vi "CRYCal Correction.vi"(4 "Calibration Response Cluster":T1={"Calibration"={"Calibration Step Name"="", "Device"="", "Correction Curve Name"="", "Equalization Curve Name"="", "Sensitivity Curve Name"="", "Corr Folder and File"="", "EQ Folder and File"="", "Sens Folder and File"="", "Corr Step size"=0, "EQ Step size"=0, "Input"=FALSE, "Last Cal Date (sec)"=timestamp(0 s since 1904-01-01), "Cha Name"="", "Corr Curve Found"=FALSE, "EQ Curve Found"=FALSE, "Sens Curve Found"=FALSE, "Signal Type"="", "Calibrated Device"="", "Hz"=0}, "Corr Curve"={"Name"="", "Curve"=[], "X data"=1, "Y data"=1, "Z data"=1, "X axis"=0, "Y axis"=1, "Z axis"=1, "X unit"="Hz", "Y unit"="", "Z unit"="deg.", "X dB ref"=1.0, "Y dB ref"=1.0, "Z dB ref"=1.0, "single val"=FALSE, "protected"=FALSE, "display X"=TRUE, "display Y"=TRUE, "display Z"=TRUE, "Test Info"="", "Step No."=0, "Plot Settings"={"Color"=0, "Interpolation"=0, "Point Style"=0, "Line Style"=0, "Point Color"=0, "Line Width"=0, "Bar Plot Style"=0, "Fill To"=0}, "AutoProtect"=FALSE}, "EQ Curve"={"Name"="", "Curve"=[], "X data"=1, "Y data"=1, "Z data"=1, "X axis"=0, "Y axis"=1, "Z axis"=1, "X unit"="Hz", "Y unit"="", "Z unit"="deg.", "X dB ref"=1.0, "Y dB ref"=1.0, "Z dB ref"=1.0, "single val"=FALSE, "protected"=FALSE, "display X"=TRUE, "display Y"=TRUE, "display Z"=TRUE, "Test Info"="", "Step No."=0, "Plot Settings"={"Color"=0, "Interpolation"=0, "Point Style"=0, "Line Style"=0, "Point Color"=0, "Line Width"=0, "Bar Plot Style"=0, "Fill To"=0}, "AutoProtect"=FALSE}, "Sens Curve"={"Name"="", "Curve"=[], "X data"=1, "Y data"=1, "Z data"=1, "X axis"=0, "Y axis"=1, "Z axis"=1, "X unit"="Hz", "Y unit"="", "Z unit"="deg.", "X dB ref"=1.0, "Y dB ref"=1.0, "Z dB ref"=1.0, "single val"=FALSE, "protected"=FALSE, "display X"=TRUE, "display Y"=TRUE, "display Z"=TRUE, "Test Info"="", "Step No."=0, "Plot Settings"={"Color"=0, "Interpolation"=0, "Point Style"=0, "Line Style"=0, "Point Color"=0, "Line Width"=0, "Bar Plot Style"=0, "Fill To"=0}, "AutoProtect"=FALSE}} {"Sens Curve"."Z data" items=["dB", "Lin"]; "Sens Curve"."X data" items=["dB", "Lin"]; "Sens Curve"."Y data" items=["dB", "Lin"]; "Sens Curve"."Z dB ref" format="%.1f"; "Sens Curve"."Z axis" items=["Log", "Lin"]; "Sens Curve"."X dB ref" format="%.1f"; "Sens Curve"."X axis" items=["Log", "Lin"]; "Sens Curve"."Y axis" items=["Log", "Lin"]; "Sens Curve"."Y dB ref" format="%.1f"; "Sens Curve"."Curve"."z" format="%.2f"; "Sens Curve"."Curve"."y" format="%.2f"; "Sens Curve"."Curve"."x" format="%.2f"; "EQ Curve"."Z data" items=["dB", "Lin"]; "EQ Curve"."X data" items=["dB", "Lin"]; "EQ Curve"."Y data" items=["dB", "Lin"]; "EQ Curve"."Z dB ref" format="%.1f"; "EQ Curve"."Z axis" items=["Log", "Lin"]; "EQ Curve"."X dB ref" format="%.1f"; "EQ Curve"."X axis" items=["Log", "Lin"]; "EQ Curve"."Y axis" items=["Log", "Lin"]; "EQ Curve"."Y dB ref" format="%.1f"; "EQ Curve"."Curve"."z" format="%.2f"; "EQ Curve"."Curve"."y" format="%.2f"; "EQ Curve"."Curve"."x" format="%.2f"; "Corr Curve"."Z data" items=["dB", "Lin"]; "Corr Curve"."X data" items=["dB", "Lin"]; "Corr Curve"."Y data" items=["dB", "Lin"]; "Corr Curve"."Z dB ref" format="%.1f"; "Corr Curve"."Z axis" items=["Log", "Lin"]; "Corr Curve"."X dB ref" format="%.1f"; "Corr Curve"."X axis" items=["Log", "Lin"]; "Corr Curve"."Y axis" items=["Log", "Lin"]; "Corr Curve"."Y dB ref" format="%.1f"; "Corr Curve"."Curve"."z" format="%.2f"; "Corr Curve"."Curve"."y" format="%.2f"; "Corr Curve"."Curve"."x" format="%.2f"; "Calibration"."EQ Step size" items=["R10", "R20", "R40", "R80", "User"]; "Calibration"."Corr Step size" items=["R10", "R20", "R40", "R80", "User"]}, 6 "Calibration Stimulus Cluster":T1={"Calibration"={"Calibration Step Name"="", "Device"="", "Correction Curve Name"="", "Equalization Curve Name"="", "Sensitivity Curve Name"="", "Corr Folder and File"="", "EQ Folder and File"="", "Sens Folder and File"="", "Corr Step size"=0, "EQ Step size"=0, "Input"=FALSE, "Last Cal Date (sec)"=timestamp(0 s since 1904-01-01), "Cha Name"="", "Corr Curve Found"=FALSE, "EQ Curve Found"=FALSE, "Sens Curve Found"=FALSE, "Signal Type"="", "Calibrated Device"="", "Hz"=0}, "Corr Curve"={"Name"="", "Curve"=[], "X data"=1, "Y data"=1, "Z data"=1, "X axis"=0, "Y axis"=1, "Z axis"=1, "X unit"="Hz", "Y unit"="", "Z unit"="deg.", "X dB ref"=1.0, "Y dB ref"=1.0, "Z dB ref"=1.0, "single val"=FALSE, "protected"=FALSE, "display X"=TRUE, "display Y"=TRUE, "display Z"=TRUE, "Test Info"="", "Step No."=0, "Plot Settings"={"Color"=0, "Interpolation"=0, "Point Style"=0, "Line Style"=0, "Point Color"=0, "Line Width"=0, "Bar Plot Style"=0, "Fill To"=0}, "AutoProtect"=FALSE}, "EQ Curve"={"Name"="", "Curve"=[], "X data"=1, "Y data"=1, "Z data"=1, "X axis"=0, "Y axis"=1, "Z axis"=1, "X unit"="Hz", "Y unit"="", "Z unit"="deg.", "X dB ref"=1.0, "Y dB ref"=1.0, "Z dB ref"=1.0, "single val"=FALSE, "protected"=FALSE, "display X"=TRUE, "display Y"=TRUE, "display Z"=TRUE, "Test Info"="", "Step No."=0, "Plot Settings"={"Color"=0, "Interpolation"=0, "Point Style"=0, "Line Style"=0, "Point Color"=0, "Line Width"=0, "Bar Plot Style"=0, "Fill To"=0}, "AutoProtect"=FALSE}, "Sens Curve"={"Name"="", "Curve"=[], "X data"=1, "Y data"=1, "Z data"=1, "X axis"=0, "Y axis"=1, "Z axis"=1, "X unit"="Hz", "Y unit"="", "Z unit"="deg.", "X dB ref"=1.0, "Y dB ref"=1.0, "Z dB ref"=1.0, "single val"=FALSE, "protected"=FALSE, "display X"=TRUE, "display Y"=TRUE, "display Z"=TRUE, "Test Info"="", "Step No."=0, "Plot Settings"={"Color"=0, "Interpolation"=0, "Point Style"=0, "Line Style"=0, "Point Color"=0, "Line Width"=0, "Bar Plot Style"=0, "Fill To"=0}, "AutoProtect"=FALSE}} {"Sens Curve"."Z data" items=["dB", "Lin"]; "Sens Curve"."X data" items=["dB", "Lin"]; "Sens Curve"."Y data" items=["dB", "Lin"]; "Sens Curve"."Z dB ref" format="%.1f"; "Sens Curve"."Z axis" items=["Log", "Lin"]; "Sens Curve"."X dB ref" format="%.1f"; "Sens Curve"."X axis" items=["Log", "Lin"]; "Sens Curve"."Y axis" items=["Log", "Lin"]; "Sens Curve"."Y dB ref" format="%.1f"; "Sens Curve"."Curve"."z" format="%.2f"; "Sens Curve"."Curve"."y" format="%.2f"; "Sens Curve"."Curve"."x" format="%.2f"; "EQ Curve"."Z data" items=["dB", "Lin"]; "EQ Curve"."X data" items=["dB", "Lin"]; "EQ Curve"."Y data" items=["dB", "Lin"]; "EQ Curve"."Z dB ref" format="%.1f"; "EQ Curve"."Z axis" items=["Log", "Lin"]; "EQ Curve"."X dB ref" format="%.1f"; "EQ Curve"."X axis" items=["Log", "Lin"]; "EQ Curve"."Y axis" items=["Log", "Lin"]; "EQ Curve"."Y dB ref" format="%.1f"; "EQ Curve"."Curve"."z" format="%.2f"; "EQ Curve"."Curve"."y" format="%.2f"; "EQ Curve"."Curve"."x" format="%.2f"; "Corr Curve"."Z data" items=["dB", "Lin"]; "Corr Curve"."X data" items=["dB", "Lin"]; "Corr Curve"."Y data" items=["dB", "Lin"]; "Corr Curve"."Z dB ref" format="%.1f"; "Corr Curve"."Z axis" items=["Log", "Lin"]; "Corr Curve"."X dB ref" format="%.1f"; "Corr Curve"."X axis" items=["Log", "Lin"]; "Corr Curve"."Y axis" items=["Log", "Lin"]; "Corr Curve"."Y dB ref" format="%.1f"; "Corr Curve"."Curve"."z" format="%.2f"; "Corr Curve"."Curve"."y" format="%.2f"; "Corr Curve"."Curve"."x" format="%.2f"; "Calibration"."EQ Step size" items=["R10", "R20", "R40", "R80", "User"]; "Calibration"."Corr Step size" items=["R10", "R20", "R40", "R80", "User"]}, 9 "Apply Corr In":bool, 10 "Apply Corr Out":bool, 11 "Frequency curve in":cluster{cluster{"x":dbl, "y":dbl, "z":dbl}[]}[](array[cluster])) -> (3 "Frequency curve out":cluster{cluster{"x":dbl, "y":dbl, "z":dbl}[]}[](array[cluster]))   [LabVIEW 2013]
uses:
  Typedef Control/CRYCalibration 2DCluster.ctl
  Typedef Control/CRYCalibration Cluster.ctl
  Typedef Control/CRYData Cluster.ctl
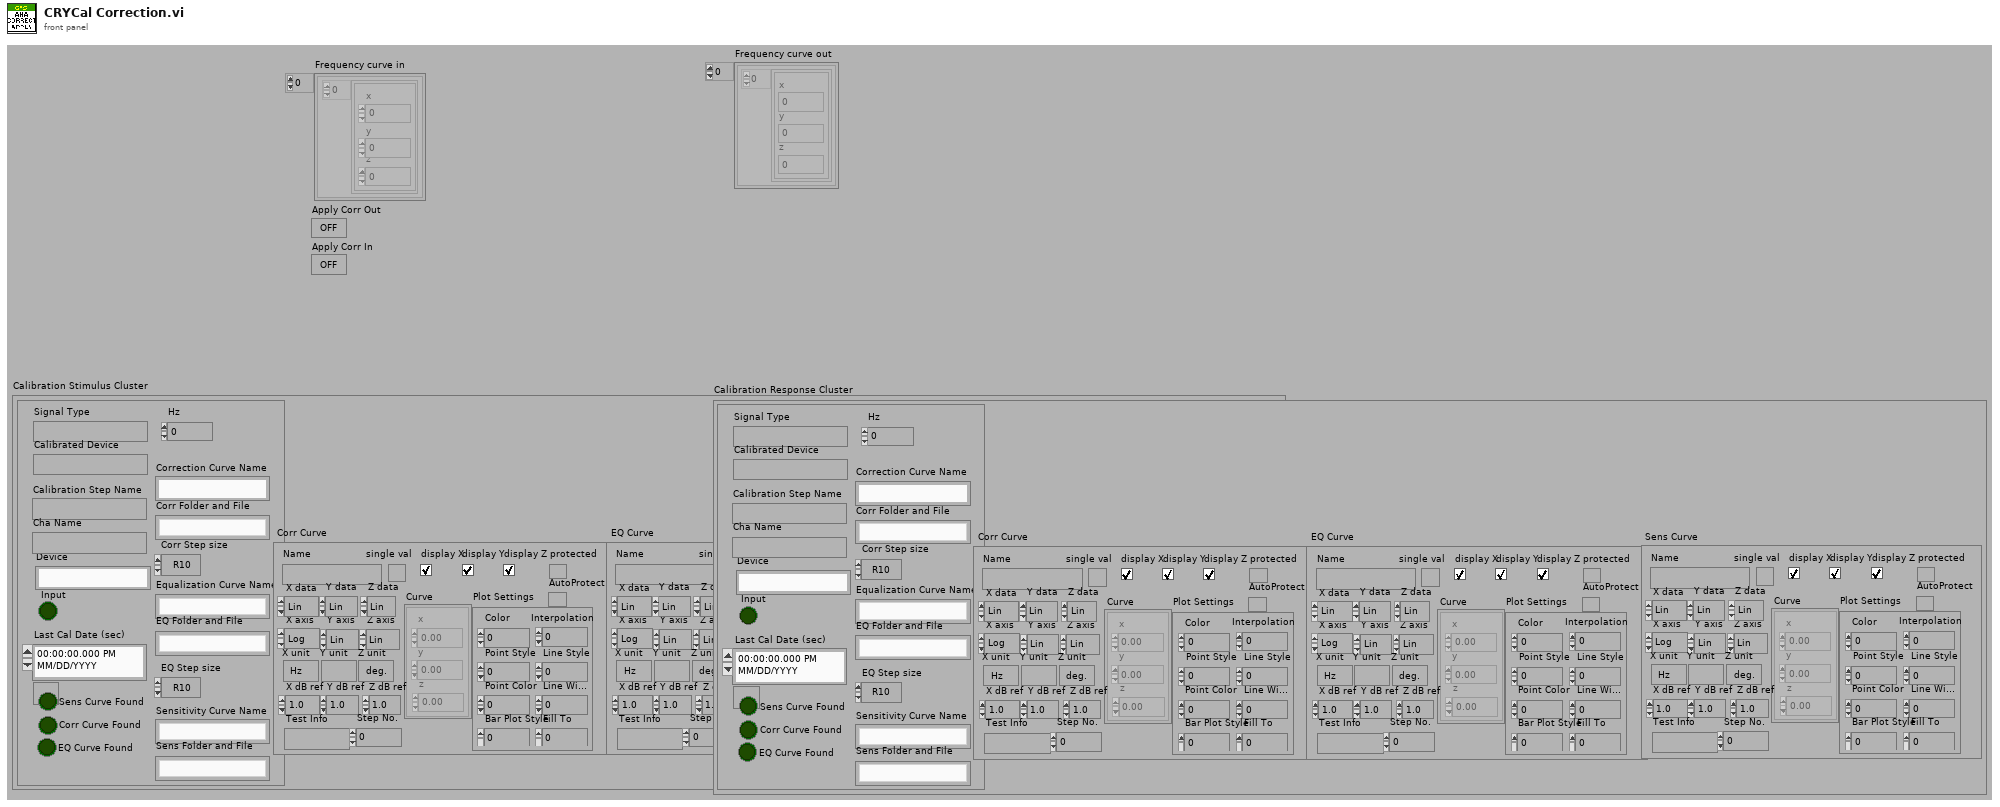
[diagram p1: front panel]
types:
  T1 = typedef "CRYCalibration 2DCluster.ctl" = cluster{"Calibration":T2, "Corr Curve":T3, "EQ Curve":T3, "Sens Curve":T3}
  T2 = typedef "CRYCalibration Cluster.ctl" = cluster{"Calibration Step Name":string, "Device":string, "Correction Curve Name":string, "Equalization Curve Name":string, "Sensitivity Curve Name":string, "Corr Folder and File":string, "EQ Folder and File":string, "Sens Folder and File":string, "Corr Step size":u16, "EQ Step size":u16, "Input":bool, "Last Cal Date (sec)":timestamp, "Cha Name":string, "Corr Curve Found":bool, "EQ Curve Found":bool, "Sens Curve Found":bool, "Signal Type":string, "Calibrated Device":string, "Hz":u32}
  T3 = typedef "CRYData Cluster.ctl" = cluster{"Name":string, "Curve":cluster{"x":dbl, "y":dbl, "z":dbl}[], "X data":u16, "Y data":u16, "Z data":u16, "X axis":u16, "Y axis":u16, "Z axis":u16, "X unit":string, "Y unit":string, "Z unit":string, "X dB ref":dbl, "Y dB ref":dbl, "Z dB ref":dbl, "single val":bool, "protected":bool, "display X":bool, "display Y":bool, "display Z":bool, "Test Info":string, "Step No.":i32, "Plot Settings":cluster{"Color":u32, "Interpolation":u8, "Point Style":u8, "Line Style":u8, "Point Color":u32, "Line Width":u8, "Bar Plot Style":u8, "Fill To":i16}, "AutoProtect":bool}
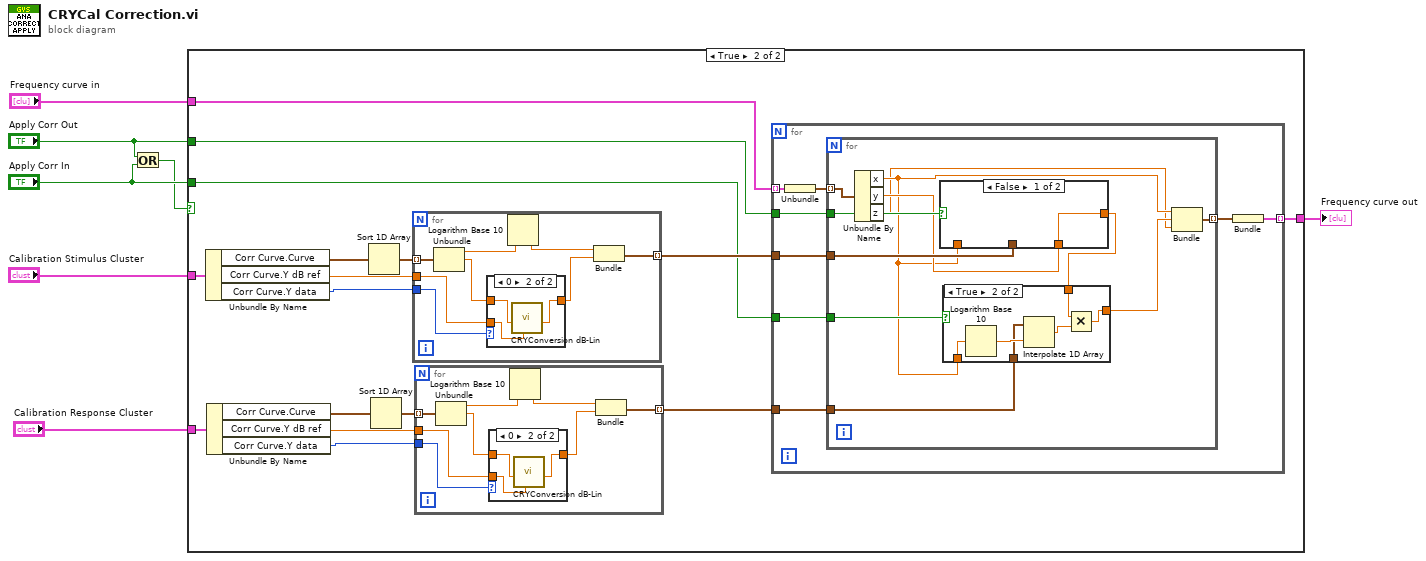
[diagram p0: block diagram]
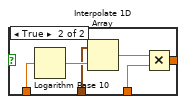
[diagram p4: hidden frame]
diagram:
  n1 = Or(x="Apply Corr Out", y="Apply Corr In") -> (x .or. y?=w3:bool)
  n2 = case shown="True" w3 {
    tunnel: "Calibration Stimulus Cluster" -> [_ w20]
    tunnel: "Calibration Response Cluster" -> [_ w15]
    tunnel: "Apply Corr Out" -> [_ w12]
    tunnel: "Apply Corr In" -> [_ w11]
    tunnel: "Frequency curve in" -> [w8 w10]
    tunnel: [w8 w9] -> w1
    frame False {
    }
    frame True {
      n3 = Unbundle By Name(w20) -> ("Corr Curve.Curve"=w23:cluster{"x":dbl, "y":dbl, "z":dbl}[], "Corr Curve.Y dB ref"=w21:dbl, "Corr Curve.Y data"=w22:u16)
      n4 = Unbundle By Name(w15) -> ("Corr Curve.Curve"=w17:cluster{"x":dbl, "y":dbl, "z":dbl}[], "Corr Curve.Y dB ref"=w19:dbl, "Corr Curve.Y data"=w18:u16)
      n5 = Sort 1D Array(array=w23) -> (sorted array=w24:cluster{"x":dbl, "y":dbl, "z":dbl}[])
      n6 = Sort 1D Array(array=w17) -> (sorted array=w16:cluster{"x":dbl, "y":dbl, "z":dbl}[])
      n7 = for {
        tunnel: w24 -> [w65] mode=indexing
        tunnel: [w63] -> w14 mode=indexing
        tunnel: w21 -> [w61]
        tunnel: w22 -> [w60]
        n8 = Unbundle(w65) -> ("x"=w59:dbl, "y"=w58:dbl)  [unwired: 1 out]
        n9 = case shown="0" w60 {
          tunnel: w58 -> [w66 w69]
          tunnel: [w66 w68] -> w62
          tunnel: w61 -> [_ w67]
          frame 1, Default {
          }
          frame 0 {
            n10 = call "CRYConversion dB-Lin.vi"("dB ref."=w67, "Log In"=w69) -> ("Lin Out"=w68:dbl)  [unwired: 4 in, 3 out]
          }
        }
        n11 = Logarithm Base 10(1:w59) -> (0:w64:dbl)
        n12 = Bundle(w64, "Lin Out"=w62) -> (w63:cluster{dbl, "Lin Out":dbl})  [unwired: 1 out]
      }
      n13 = for {
        tunnel: w16 -> [w77] mode=indexing
        tunnel: [w75] -> w13 mode=indexing
        tunnel: w19 -> [w73]
        tunnel: w18 -> [w72]
        n14 = Unbundle(w77) -> ("x"=w71:dbl, "y"=w70:dbl)  [unwired: 1 out]
        n15 = case shown="0" w72 {
          tunnel: w70 -> [w78 w81]
          tunnel: [w78 w80] -> w74
          tunnel: w73 -> [_ w79]
          frame 1, Default {
          }
          frame 0 {
            n16 = call "CRYConversion dB-Lin.vi"("dB ref."=w79, "Log In"=w81) -> ("Lin Out"=w80:dbl)  [unwired: 4 in, 3 out]
          }
        }
        n17 = Logarithm Base 10(1:w71) -> (0:w76:dbl)
        n18 = Bundle(w76, "Lin Out"=w74) -> (w75:cluster{dbl, "Lin Out":dbl})  [unwired: 1 out]
      }
      n19 = for {
        tunnel: w14 -> [w32]
        tunnel: w13 -> [w31]
        tunnel: w12 -> [w30]
        tunnel: w11 -> [w29]
        tunnel: w10 -> [w28] mode=indexing
        tunnel: [w25] -> w9 mode=indexing
        n20 = Unbundle(w28) -> (w27:cluster{"x":dbl, "y":dbl, "z":dbl}[])
        n21 = for {
          tunnel: w32 -> [w43]
          tunnel: w31 -> [w42]
          tunnel: w30 -> [w41]
          tunnel: w29 -> [w40]
          tunnel: w27 -> [w38] mode=indexing
          tunnel: [w33] -> w26 mode=indexing
          n22 = Unbundle By Name(w38) -> ("x"=w35:dbl, "y"=w37:dbl, "z"=w34:dbl)
          n23 = case shown="False" w41 {
            tunnel: w43 -> [_ w55]
            tunnel: w37 -> [w51 w54]
            tunnel: w35 -> [_ w53]
            tunnel: [w51 w52] -> w39
            frame False {
            }
            frame True {
              n24 = Logarithm Base 10(1:w53) -> (0:w57:dbl)
              n25 = Interpolate 1D Array(1:w57, 2:w55) -> (0:w56:dbl)
              n26 = Multiply(x=w56, y=w54) -> (x*y=w52:dbl)
            }
          }
          n27 = case shown="True" w40 {
            tunnel: w42 -> [_ w45]
            tunnel: w35 -> [_ w48]
            tunnel: w39 -> [w44 w47]
            tunnel: [w44 w46] -> w36
            frame False {
            }
            frame True {
              n28 = Logarithm Base 10(1:w48) -> (0:w50:dbl)
              n29 = Interpolate 1D Array(1:w50, 2:w45) -> (0:w49:dbl)
              n30 = Multiply(x=w47, y=w49) -> (x*y=w46:dbl)
            }
          }
          n31 = Bundle("x"=w35, "y"=w36, "z"=w34) -> (w33:cluster{"x":dbl, "y":dbl, "z":dbl})  [unwired: 1 in]
        }
        n32 = Bundle(w26) -> (w25:cluster{cluster{"x":dbl, "y":dbl, "z":dbl}[]})  [unwired: 1 in]
      }
    }
  }
  "Frequency curve out" <- w1
